vi "WSVCAP SHL Host LL Interface Core.vi"(0 "Message In":string, 11 "error in":errorcluster, 12 "Log (T)":bool=TRUE, 13 "Function":T5, 14 "FPGA":T1) -> (3 "System":T2={"Settings"={"I2C Slave Address"=144, "I2C Clock Rate (Hz)"=20.0, "SPI Clock Rate (Hz)"=50000.0, "RFFE Slave Address"=255, "RFFE Clock Rate (Hz)"=20.0, "Simulate FPGA"=TRUE, "C1 Cap DAC Default"=165, "C2 Cap DAC Default"=165, "C3 Cap DAC Default"=134, "C4 Cap DAC Default"=150}, "FPGA Resource"="", "Online"=FALSE, "I2C Wait Ticks"=0, "SPI Wait Ticks"=0, "RFFE Wait Ticks"=0, "FPGA VI Reference (FPGA Mode)"=refnum, "FPGA VI Reference (Sim Mode)"=refnum} {"Settings"."C4 Cap DAC Default" format="0x%02x"; "Settings"."C3 Cap DAC Default" format="0x%02x"; "Settings"."C2 Cap DAC Default" format="0x%02x"; "Settings"."C1 Cap DAC Default" format="0x%02x"; "Settings"."RFFE Clock Rate (Hz)" format="%.0f Hz"; "Settings"."RFFE Slave Address" format="0x%02x"; "Settings"."I2C Clock Rate (Hz)" format="%.0f Hz"; "Settings"."SPI Clock Rate (Hz)" format="%.0f Hz"; "Settings"."I2C Slave Address" format="0x%02x"}, 4 "Message Out":string, 15 "error out":errorcluster)   [LabVIEW 2017]
uses:
  Type Defs/WSVCAP SHL Function Enum.ctl
  Type Defs/WSVCAP SHL Core System Cluster.ctl
  Type Defs/WSVCAP SHL I2C Settings Cluster.ctl
  Type Defs/WSVCAP SHL FPGA Ref.ctl
  Type Defs/WSVCAP SHL FPGA Enum.ctl
  user.lib/Utilities/Type Defs/MISC IO Choice Enum.ctl
  Type Defs/WSVCAP SHL Gatekeeper Operation Enum.ctl
  user.lib/Configuration Files/Type Defs/CFG File Operation Enum.ctl
  Type Defs/WSVCAP SHL Top Level Control Enum.ctl
  <vilib>/FPGAPlugInAG/PXI-7813R/niLvFpga_Open_PXI-7813R.vi
  <vilib>/FPGAPlugInAG/PXI-7813R/niLvFpga_Reset_PXI-7813R.vi
  <vilib>/FPGAPlugInAG/PXI-7813R/niLvFpga_Run_PXI-7813R.vi
  <vilib>/FPGAPlugInAG/PXI-7813R/niLvFpga_Abort_PXI-7813R.vi
  <vilib>/FPGAPlugInAG/PXI-7813R/niLvFpga_Close_PXI-7813R.vi
  <vilib>/rvi/interface/nirviOpenFPGA/nirviOpenFPGA.xnode
  FPGA Bitfiles/WSVCAPShell_WiSpryFPGA1_WSVCAPSHLFPGATLT_ffr+nD2N+rA.lvbitx
  <vilib>/rvi/interface/nirviMethod/nirviMethod.xnode
  <vilib>/rvi/interface/nirviCloseFPGA/nirviCloseFPGA.xnode
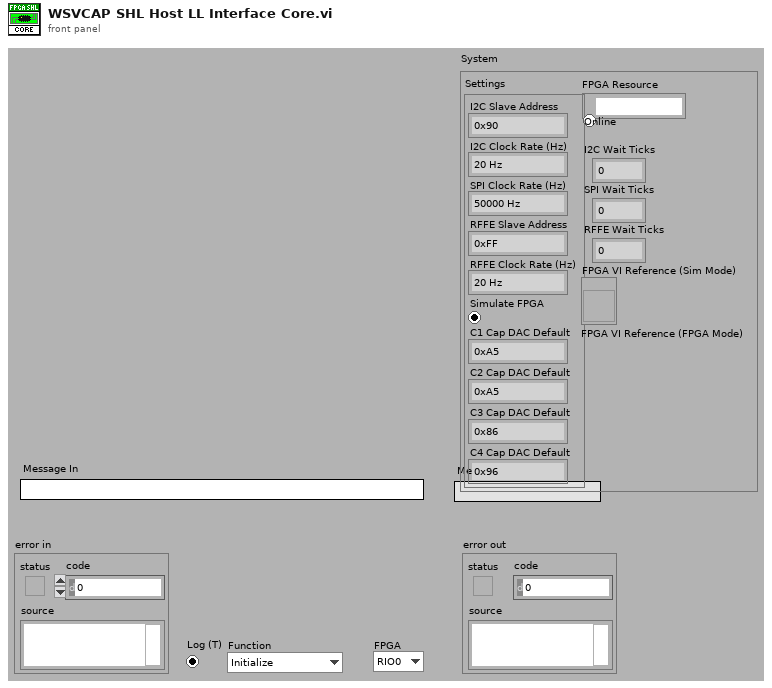
[diagram p1: front panel]
types:
  T1 = typedef "WSVCAP SHL FPGA Enum.ctl" = enum16{"RIO0", "RIO1"}
  T2 = typedef "WSVCAP SHL Core System Cluster.ctl" = cluster{"Settings":T3, "FPGA Resource":tag, "Online":bool, "I2C Wait Ticks":u32, "SPI Wait Ticks":u32, "RFFE Wait Ticks":u32, "FPGA VI Reference (FPGA Mode)":T4, "FPGA VI Reference (Sim Mode)":refnum<vi>}
  T3 = typedef "WSVCAP SHL I2C Settings Cluster.ctl" = cluster{"I2C Slave Address":u8, "I2C Clock Rate (Hz)":dbl, "SPI Clock Rate (Hz)":dbl, "RFFE Slave Address":u8, "RFFE Clock Rate (Hz)":dbl, "Simulate FPGA":bool, "C1 Cap DAC Default":u8, "C2 Cap DAC Default":u8, "C3 Cap DAC Default":u8, "C4 Cap DAC Default":u8}
  T4 = typedef "WSVCAP SHL FPGA Ref.ctl" = refnum<k20>
  T5 = typedef "WSVCAP SHL Function Enum.ctl" = enum16{"Initialize", "Configure I2C", "Configure RFFE", "Write I2C", "Read I2C", "Write RFFE", "Read RFFE", "Start RFFE Cycle", "Stop RFFE Cycle", "Get Status", "Close"}
  T6 = typedef "WSVCAP SHL Gatekeeper Operation Enum.ctl" = enum16{"Initialize", "Lock", "Unlock", "Close"}
  T7 = typedef "MISC IO Choice Enum.ctl" = enum16{"Read", "Write"}
  T8 = typedef "CFG File Operation Enum.ctl" = enum16{"Read", "Write", "Copy", "Edit"}
  T9 = enum32{"Invalid", "Standard", "Closed", "Hidden", "Minimized", "Maximized"}
  T10 = typedef "WSVCAP SHL Top Level Control Enum.ctl" = enum16{"Start", "Cmd", "Transaction", "Wait Ticks", "Socket Mask", "UUT Set", "Slave Address", "Sub Address", "Bytes to Write", "Bytes to Read", "Write Data", "Write Flag", "Read Data", "Read Flag", "Ack Read", "Read Status Flag", "Ack Read Status", "Status", "Cycle Count", "Stop Cycle", "Exit"}
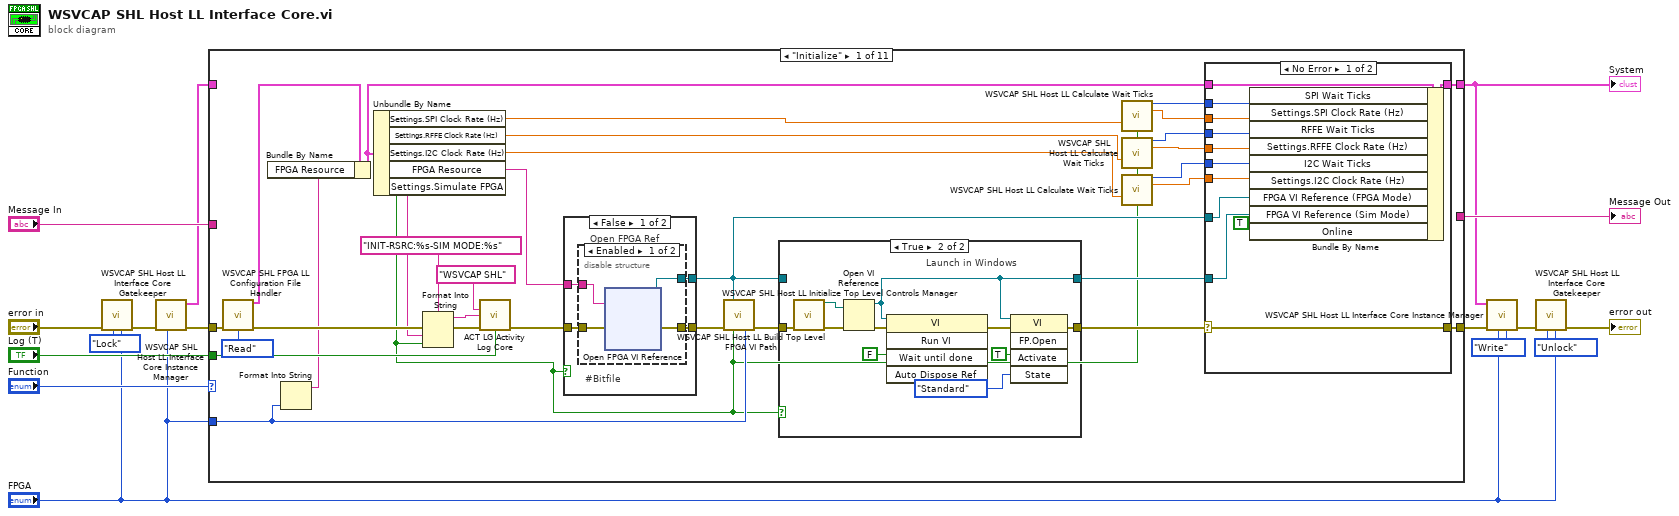
[diagram p0: block diagram]
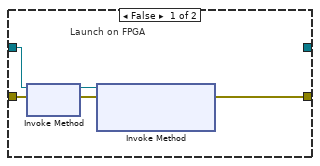
[diagram p4: hidden frame]
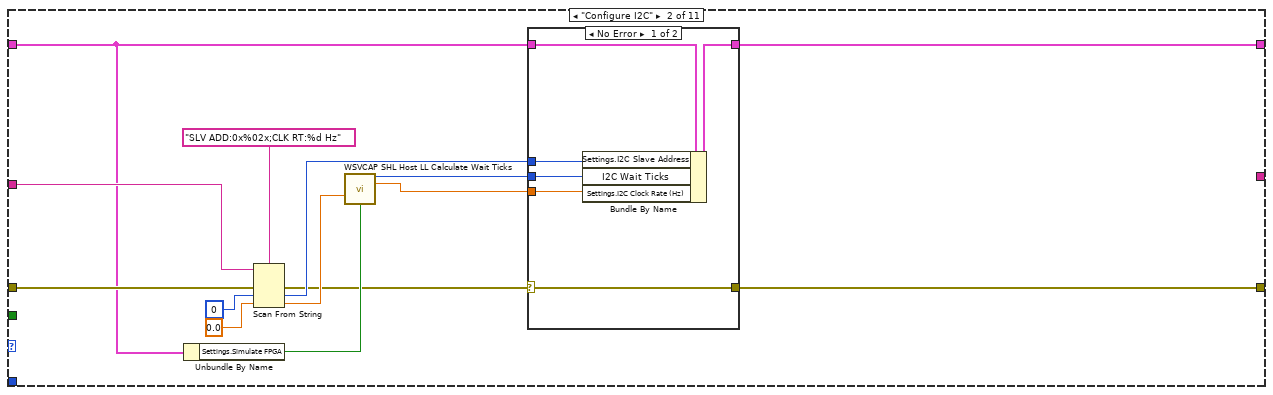
[diagram p6: hidden frame]
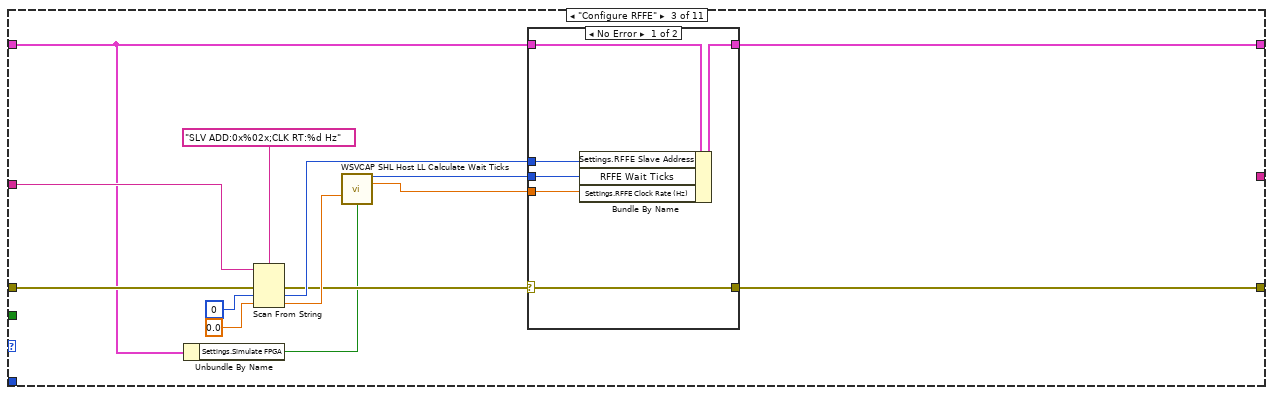
[diagram p8: hidden frame]
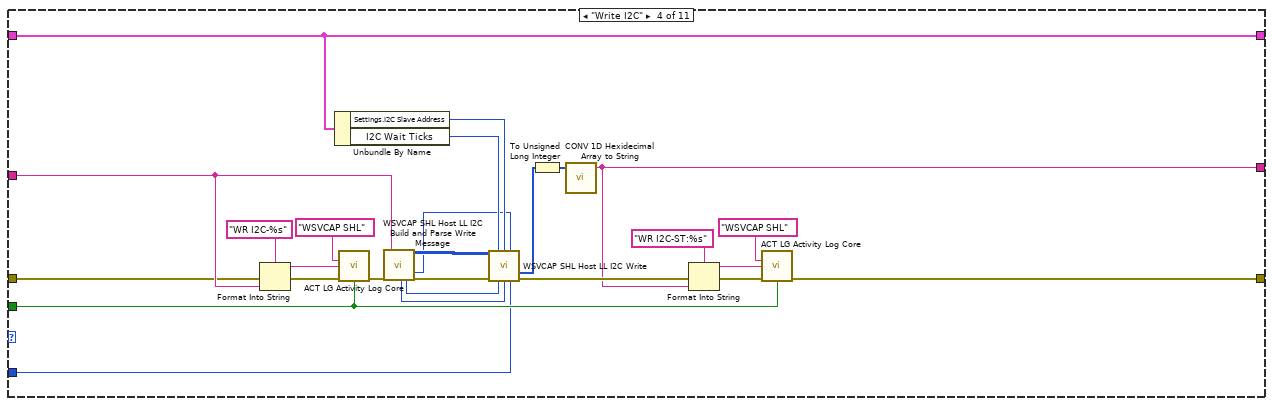
[diagram p10: hidden frame]
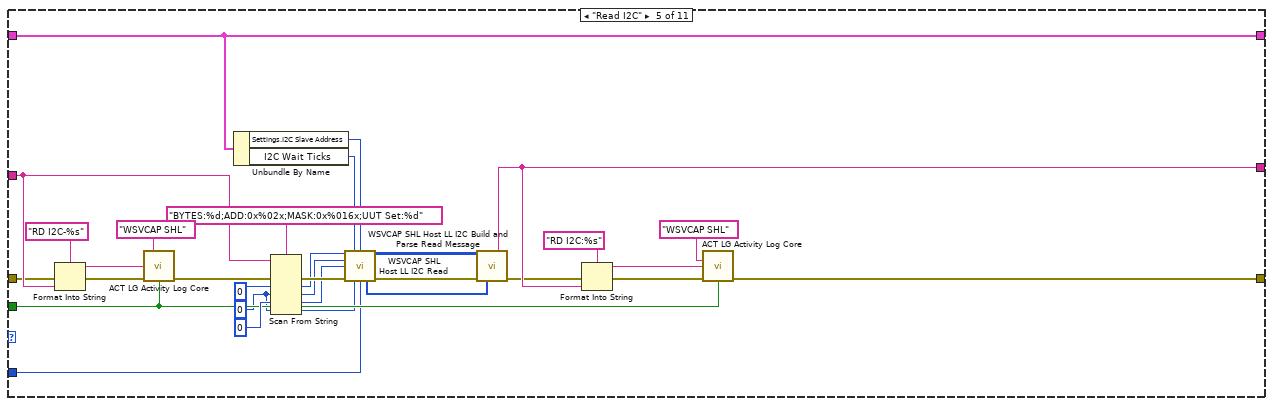
[diagram p11: hidden frame]
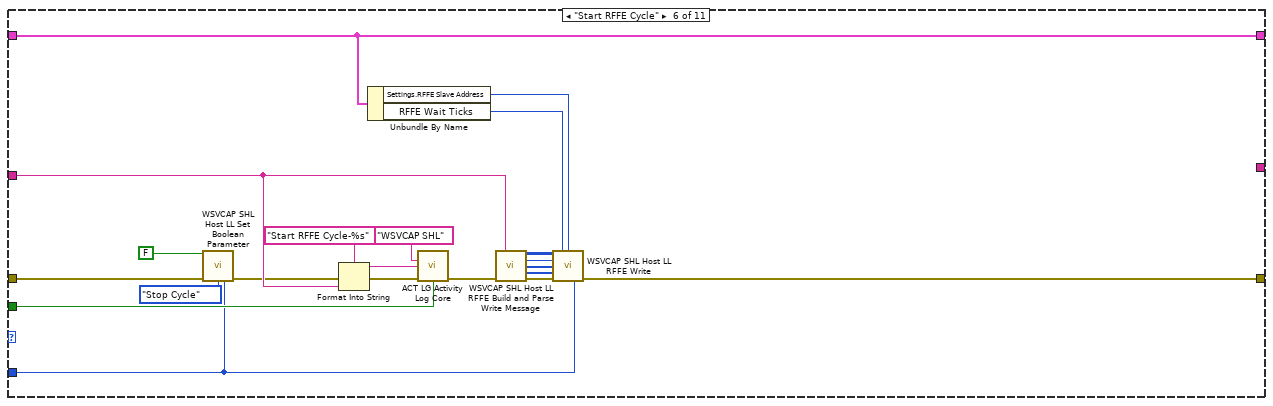
[diagram p12: hidden frame]
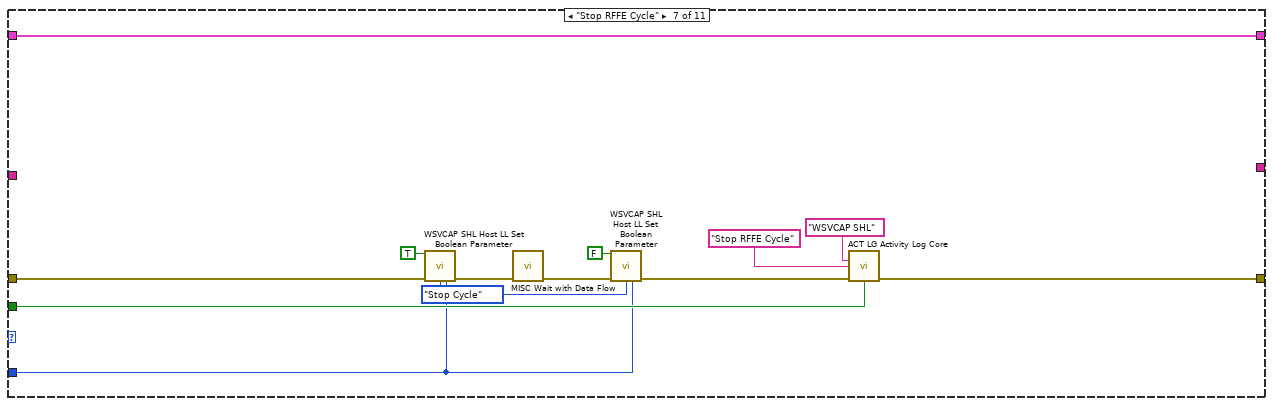
[diagram p13: hidden frame]
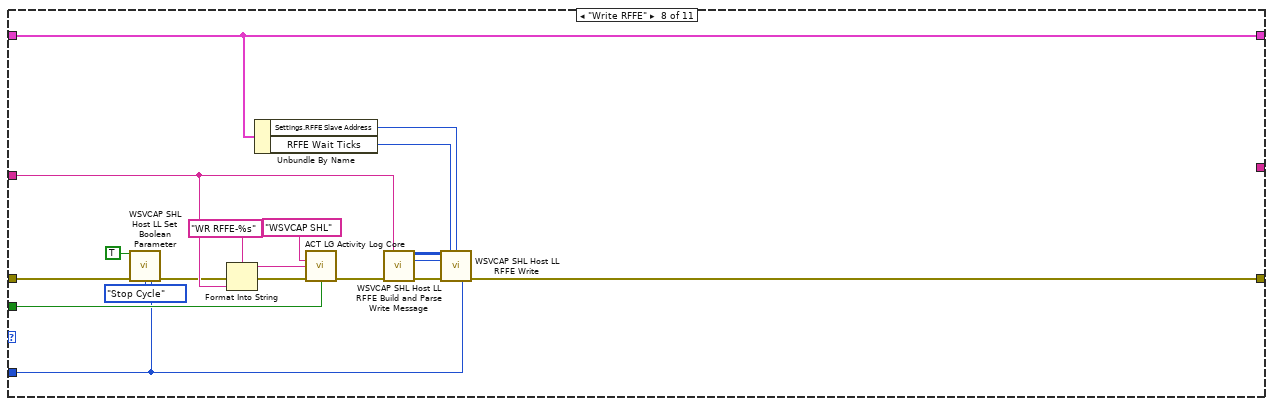
[diagram p14: hidden frame]
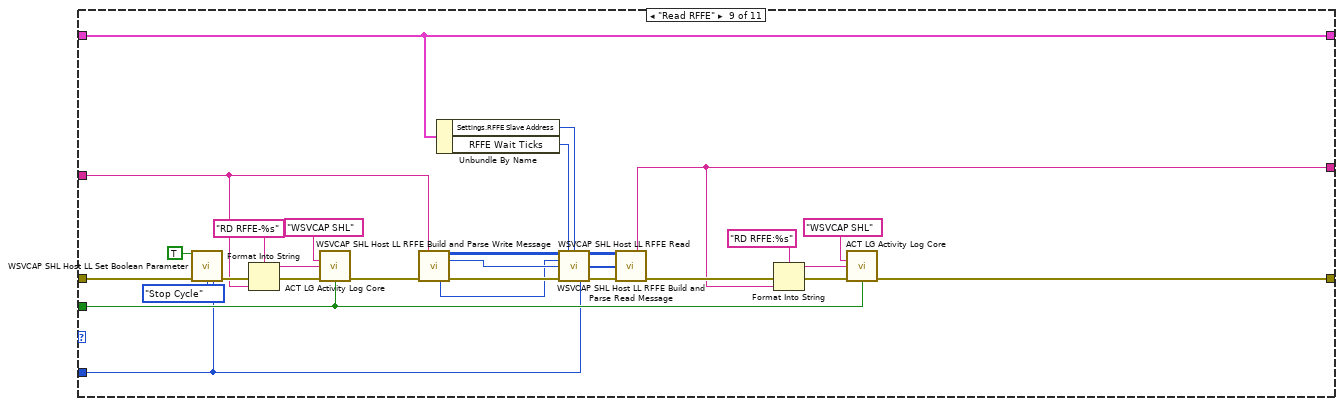
[diagram p15: hidden frame]
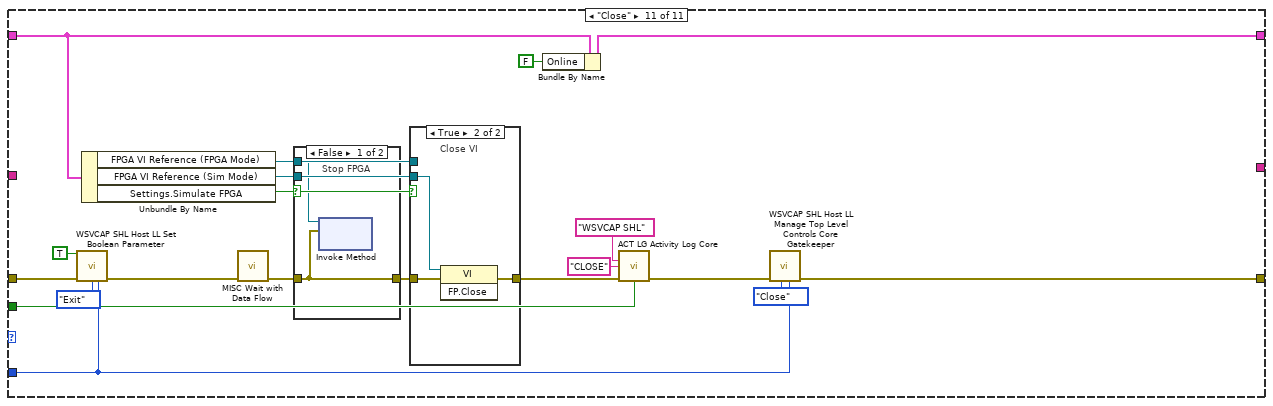
[diagram p17: hidden frame]
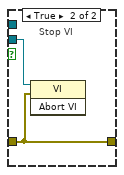
[diagram p18: hidden frame]
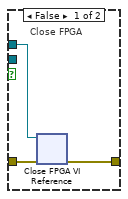
[diagram p19: hidden frame]
diagram:
  n1 = call "WSVCAP SHL Host LL Interface Core Gatekeeper.vi"("FPGA"="FPGA", "Operation"=WSVCAP_SHL_Gatekeeper_Operation_Enum."Lock", "error in (no error)"="error in") -> ("error out"=w4:errorcluster)  [unwired: 8 in]
  n2 = call "WSVCAP SHL Host LL Interface Core Instance Manager.vi"("FPGA"="FPGA", "error in (no error)"=w4) -> ("error out"=w10:errorcluster, "FGPA Interface Out"=w9:T2)  [unwired: 8 in]
  n3 = case shown="\"Initialize\"" "Function" {
    tunnel: w10 -> [w43 w98 w120 w149 w170 w190 w216 w230 w253 w270 w288]
    tunnel: "Message In" -> [_ w97 w119 w150 w171 w201 _ w233 w246 _ _]
    tunnel: [w46 w99 w121 w151 w167 w199 w219 w225 w257 w270 w273] -> w12
    tunnel: [w47 w100 w122 w137 w163 w195 w221 w227 w251 w271 w291] -> w11
    tunnel: w9 -> [_ w93 w115 w137 w163 w195 w221 w227 w251 w271 w281]
    tunnel: [_ _ _ w141 w172 _ _ _ w256 _ _] -> w14
    tunnel: "Log (T)" -> [w36 _ _ w138 w164 w200 w218 w232 w255 _ w284]
    tunnel: "FPGA" -> [w20 _ _ w132 w158 w188 w214 w223 w242 _ w272]
    frame "Initialize" {
      n4 = call "WSVCAP SHL FPGA LL Configuration File Handler.vi"("Error In (no error)"=w43, "Operation"=CFG_File_Operation_Enum."Read") -> ("Object Cluster Out"=w23:T2, "Error Out"=w41:errorcluster)  [unwired: 11 in, 1 out]
      n5 = Format Into String(w20) -> (resulting string=w24:string)  [unwired: 3 in, 1 out]
      n6 = Bundle By Name(cluster=w23, "FPGA Resource"=w24) -> (w22:T2)
      n7 = Unbundle By Name(w22) -> ("Settings.SPI Clock Rate (Hz)"=w31:dbl, "Settings.RFFE Clock Rate (Hz)"=w34:dbl, "Settings.I2C Clock Rate (Hz)"=w38:dbl, "FPGA Resource"=w28:tag, "Settings.Simulate FPGA"=w19:bool)
      n8 = Format Into String(format string="INIT-RSRC:%s-SIM MODE:%s", error in=w41, w28, w19) -> (resulting string=w42:string, error out=w40:errorcluster)  [unwired: 1 in]
      n9 = call "ACT LG Activity Log Core.vi"("Source"="WSVCAP SHL", "Log Line"=w42, "Error In (no error)"=w40, "Log (T)"=w36) -> ("Error Out"=w27:errorcluster)  [unwired: 10 in, 1 out]
      n10 = case shown="False" w19 {
        tunnel: [w51 w57] -> w18
        tunnel: w27 -> [w50 w57]
        tunnel: [w49 _] -> w21
        tunnel: w28 -> [w48 _]
        frame False {
          # "#Bitfile"
          # "Open FPGA Ref"
          n11 = disable-structure shown="Enabled" {
            disable-tunnel: w50 -> [w55 w56]
            disable-tunnel: [w54 w56] -> w51
            disable-tunnel: [w53 _] -> w49
            disable-tunnel: w48 -> [w52 _]
            frame Enabled {
              n12 = xnode "Open FPGA VI Reference"("error in"=w55, "resource name"=w52) -> ("FPGA VI Reference Out"=w53:T4, "error out"=w54:errorcluster)
            }
            frame Disabled {
            }
          }
        }
        frame True {
          # "Simulate FPGA"
        }
      }
      n13 = call "WSVCAP SHL Host LL Initialize Top Level Controls Manager.vi"("FPGA VI Reference (Init Only)"=w21, "error in (no error)"=w18, "Simulate FPGA (Init Only)"=w19, "FPGA"=w20) -> ("error out"=w17:errorcluster)  [unwired: 11 in]
      n14 = case shown="True" w19 {
        tunnel: w17 -> [w61 w65]
        tunnel: [w60 w68] -> w26
        tunnel: w21 -> [w58 _]
        tunnel: [_ w69] -> w25
        frame False {
          # "Launch on FPGA"
          n15 = xnode "Invoke Method"("FPGA VI Reference In"=w58, "error in"=w61) -> ("FPGA VI Reference Out"=w59:T4, "error out"=w62:errorcluster)
          n16 = xnode "Invoke Method"("FPGA VI Reference In"=w59, "error in"=w62) -> ("error out"=w60:errorcluster)  [unwired: 1 in, 1 out]
        }
        frame True {
          # "Launch in Windows"
          n17 = call "WSVCAP SHL Host LL Build Top Level FPGA VI Path.vi"("Error In (no error)"=w65) -> ("Top Level FPGA VI Path"=w63:path, "Error Out"=w64:errorcluster)  [unwired: 13 in]
          n18 = Open VI Reference(vi path=w63, error in (no error)=w64) -> (vi reference=w69:refnum<vi>, error out=w72:errorcluster)  [unwired: 4 in]
          n19 = invoke class="VI" method="Run VI"(reference=w69, error in=w72, "Wait until done"=FALSE ("Wait Until Done")) -> (error out=w70:errorcluster)  [unwired: 2 in, 4 out]
          n20 = invoke class="VI" method="FP.Open"(reference=w69, error in=w70, "Activate"=TRUE ("Activate?"), "State"=T9."Standard" ("Front Panel Window:State")) -> (error out=w68:errorcluster)  [unwired: 1 in, 4 out]
        }
      }
      n21 = call "WSVCAP SHL Host LL Calculate Wait Ticks.vi"("Clock Rate (Hz)"=w31, "Simulate FPGA"=w19) -> ("Wait Ticks"=w30:u32, "Actual Rate (Hz)"=w29:dbl)  [unwired: 12 in]
      n22 = call "WSVCAP SHL Host LL Calculate Wait Ticks.vi"("Clock Rate (Hz)"=w34, "Simulate FPGA"=w19) -> ("Wait Ticks"=w33:u32, "Actual Rate (Hz)"=w32:dbl)  [unwired: 12 in]
      n23 = call "WSVCAP SHL Host LL Calculate Wait Ticks.vi"("Clock Rate (Hz)"=w38, "Simulate FPGA"=w19) -> ("Wait Ticks"=w35:u32, "Actual Rate (Hz)"=w45:dbl)  [unwired: 12 in]
      n24 = case shown="No Error" w26 {
        selector: w26 -> [w82 w85]
        tunnel: w22 -> [w84 w86]
        tunnel: [w83 w86] -> w47
        tunnel: [w82 w85] -> w46
        tunnel: w45 -> [w81 _]
        tunnel: w35 -> [w80 _]
        tunnel: w33 -> [w79 _]
        tunnel: w32 -> [w78 _]
        tunnel: w30 -> [w77 _]
        tunnel: w29 -> [w76 _]
        tunnel: w21 -> [w74 _]
        tunnel: w25 -> [w73 _]
        frame No Error {
          n25 = Bundle By Name(cluster=w84, "SPI Wait Ticks"=w77, "Settings.SPI Clock Rate (Hz)"=w76, "RFFE Wait Ticks"=w79, "Settings.RFFE Clock Rate (Hz)"=w78, "I2C Wait Ticks"=w80, "Settings.I2C Clock Rate (Hz)"=w81, "FPGA VI Reference (FPGA Mode)"=w74, "FPGA VI Reference (Sim Mode)"=w73, "Online"=TRUE) -> (w83:T2)
        }
        frame Error {
        }
      }
    }
    frame "Configure I2C" {
      n26 = Unbundle By Name(w93) -> ("Settings.Simulate FPGA"=w92:bool)
      n27 = Scan From String(format string="SLV ADD:0x%02x;CLK RT:%d Hz", input string=w97, error in=w98, default 1=u8 0 ("I2C_Slave Address"), default 2=0.0 ("Clock Rate (Hz)")) -> (error out=w87:errorcluster, output 1=w94:u8, output 2=w90:dbl)  [unwired: 1 in, 2 out]
      n28 = call "WSVCAP SHL Host LL Calculate Wait Ticks.vi"("Clock Rate (Hz)"=w90, "Simulate FPGA"=w92) -> ("Wait Ticks"=w88:u32, "Actual Rate (Hz)"=w89:dbl)  [unwired: 12 in]
      n29 = case shown="No Error" w87 {
        selector: w87 -> [w104 w107]
        tunnel: w93 -> [w106 w108]
        tunnel: [w105 w108] -> w100
        tunnel: [w104 w107] -> w99
        tunnel: w94 -> [w103 _]
        tunnel: w89 -> [w102 _]
        tunnel: w88 -> [w101 _]
        frame No Error {
          n30 = Bundle By Name(cluster=w106, "Settings.I2C Slave Address"=w103, "I2C Wait Ticks"=w101, "Settings.I2C Clock Rate (Hz)"=w102) -> (w105:T2)
        }
        frame Error {
        }
      }
    }
    frame "Configure RFFE" {
      n31 = Unbundle By Name(w115) -> ("Settings.Simulate FPGA"=w109:bool)
      n32 = Scan From String(format string="SLV ADD:0x%02x;CLK RT:%d Hz", input string=w119, error in=w120, default 1=u8 0 ("I2C_Slave Address"), default 2=0.0 ("Clock Rate (Hz)")) -> (error out=w110:errorcluster, output 1=w116:u8, output 2=w113:dbl)  [unwired: 1 in, 2 out]
      n33 = call "WSVCAP SHL Host LL Calculate Wait Ticks.vi"("Clock Rate (Hz)"=w113, "Simulate FPGA"=w109) -> ("Wait Ticks"=w112:u32, "Actual Rate (Hz)"=w111:dbl)  [unwired: 12 in]
      n34 = case shown="No Error" w110 {
        selector: w110 -> [w126 w129]
        tunnel: w115 -> [w128 w130]
        tunnel: [w127 w130] -> w122
        tunnel: [w126 w129] -> w121
        tunnel: w116 -> [w125 _]
        tunnel: w111 -> [w124 _]
        tunnel: w112 -> [w123 _]
        frame No Error {
          n35 = Bundle By Name(cluster=w128, "Settings.RFFE Slave Address"=w125, "RFFE Wait Ticks"=w123, "Settings.RFFE Clock Rate (Hz)"=w124) -> (w127:T2)
        }
        frame Error {
        }
      }
    }
    frame "Write I2C" {
      n36 = Format Into String(format string="WR I2C-%s", error in=w149, w150) -> (resulting string=w146:string, error out=w148:errorcluster)  [unwired: 1 in]
      n37 = Unbundle By Name(w137) -> ("Settings.I2C Slave Address"=w134:u8, "I2C Wait Ticks"=w136:u32)
      n38 = call "ACT LG Activity Log Core.vi"("Source"="WSVCAP SHL", "Log Line"=w146, "Error In (no error)"=w148, "Log (T)"=w138) -> ("Error Out"=w153:errorcluster)  [unwired: 10 in, 1 out]
      n39 = call "WSVCAP SHL Host LL I2C Build and Parse Write Message.vi"("error in"=w153, "Message In"=w150) -> ("UUT Set (0/1) Out (Legacy)"=w133:u8, "Sub Address Out"=w135:u8, "C Write Data Out [DUT Ordered]"=w155:u8[][], "Socket Mask [U64] Out"=w131:u64, "error out"=w156:errorcluster)  [unwired: 12 in, 1 out]
      n40 = call "WSVCAP SHL Host LL I2C Write.vi"("C1 Data Out [DUT Ordered]"=w155, "Wait Ticks"=w136, "Slave Address"=w134, "Socket Mask [U64]"=w131, "error in"=w156, "Sub Address"=w135, "UUT Set (0/1)"=w133, "FPGA"=w132) -> ("Status"=w143:u8[], "error out"=w145:errorcluster)  [unwired: 6 in]
      n41 = To Unsigned Long Integer(number=w143) -> (unsigned 32bit integer=w142:u32[])
      n42 = call "CONV 1D Hexidecimal Array to String.vi"("1-D Hexidecimal"=w142) -> ("String"=w141:string)  [unwired: 8 in]
      n43 = Format Into String(format string="WR I2C-ST:%s", error in=w145, w141) -> (resulting string=w139:string, error out=w144:errorcluster)  [unwired: 1 in]
      n44 = call "ACT LG Activity Log Core.vi"("Source"="WSVCAP SHL", "Log Line"=w139, "Error In (no error)"=w144, "Log (T)"=w138) -> ("Error Out"=w151:errorcluster)  [unwired: 10 in, 1 out]
    }
    frame "Read I2C" {
      w160 = u8 0 ("Sub Address [U8]")
      n45 = Format Into String(format string="RD I2C-%s", error in=w170, w171) -> (resulting string=w176:string, error out=w178:errorcluster)  [unwired: 1 in]
      n46 = call "ACT LG Activity Log Core.vi"("Source"="WSVCAP SHL", "Log Line"=w176, "Error In (no error)"=w178, "Log (T)"=w164) -> ("Error Out"=w169:errorcluster)  [unwired: 10 in, 1 out]
      n47 = Unbundle By Name(w163) -> ("Settings.I2C Slave Address"=w161:u8, "I2C Wait Ticks"=w162:u32)
      n48 = Scan From String(format string="BYTES:%d;ADD:0x%02x;MASK:0x%016x;UUT Set:%d", input string=w171, error in=w169, default 1=u8 0 ("Bytes to Read"), default 2=w160, default 3=u64 0 ("Socket Mask [U32]"), default 4=w160) -> (error out=w187:errorcluster, output 1=w184:u8, output 2=w182:u8, output 3=w183:u64, output 4=w159:u8)  [unwired: 1 in, 2 out]
      n49 = call "WSVCAP SHL Host LL I2C Read.vi"("Bytes to Read"=w184, "Wait Ticks"=w162, "Slave Address"=w161, "Sub Address [U8]"=w182, "Socket Mask [U64]"=w183, "error in"=w187, "UUT Set (0/1)"=w159, "FPGA"=w158) -> ("C1:1-12 Read Data"=w180:u8[][], "Status"=w157:u8[], "error out"=w181:errorcluster)  [unwired: 5 in]
      n50 = call "WSVCAP SHL Host LL I2C Build and Parse Read Message.vi"("C1 Read Data In"=w180, "error in"=w181, "Status In"=w157) -> ("Message Out"=w172:string, "error out"=w168:errorcluster)  [unwired: 9 in, 2 out]
      n51 = Format Into String(format string="RD I2C:%s", error in=w168, w172) -> (resulting string=w173:string, error out=w175:errorcluster)  [unwired: 1 in]
      n52 = call "ACT LG Activity Log Core.vi"("Source"="WSVCAP SHL", "Log Line"=w173, "Error In (no error)"=w175, "Log (T)"=w164) -> ("Error Out"=w167:errorcluster)  [unwired: 10 in, 1 out]
    }
    frame "Start RFFE Cycle" {
      n53 = call "WSVCAP SHL Host LL Set Boolean Parameter.vi"("Boolean In"=FALSE ("Cycle (F:Write/Read - T:Write Only - No Read)"), "error in (no error)"=w190, "FPGA Top Level Control"=WSVCAP_SHL_Top_Level_Control_Enum."Stop Cycle", "FPGA"=w188) -> ("error out"=w189:errorcluster)  [unwired: 11 in]
      n54 = Format Into String(format string="Start RFFE Cycle-%s", error in=w189, w201) -> (resulting string=w203:string, error out=w205:errorcluster)  [unwired: 1 in]
      n55 = Unbundle By Name(w195) -> ("Settings.RFFE Slave Address"=w193:u8, "RFFE Wait Ticks"=w194:u32)
      n56 = call "ACT LG Activity Log Core.vi"("Source"="WSVCAP SHL", "Log Line"=w203, "Error In (no error)"=w205, "Log (T)"=w200) -> ("Error Out"=w202:errorcluster)  [unwired: 10 in, 1 out]
      n57 = call "WSVCAP SHL Host LL RFFE Build and Parse Write Message.vi"("Message In"=w201, "error in"=w202) -> ("Write Data Out [DUT Ordered]"=w207:u8[][], "Socket Mask [U16] Out"=w198:u64, "Cycle CMD Lengths Out (bits)"=w197:u8[], "Cycle CMD Delay Out (ticks)"=w196:u32[], "error out"=w208:errorcluster)  [unwired: 7 in, 2 out]
      n58 = call "WSVCAP SHL Host LL RFFE Write.vi"("RTFFE Data"=w207, "Wait Ticks"=w194, "Slave Address"=w193, "Socket Mask"=w198, "Cycle CMD Lengths Out (bits)"=w197, "Cycle CMD Delay Out (ticks)"=w196, "error in"=w208, "FPGA"=w188) -> ("error out"=w199:errorcluster)  [unwired: 6 in, 1 out]
    }
    frame "Stop RFFE Cycle" {
      w213 = WSVCAP_SHL_Top_Level_Control_Enum."Stop Cycle" ("FPGA Top Level Control")
      n59 = call "WSVCAP SHL Host LL Set Boolean Parameter.vi"("Boolean In"=TRUE ("Cycle (F:Write/Read - T:Write Only - No Read)"), "error in (no error)"=w216, "FPGA Top Level Control"=w213, "FPGA"=w214) -> ("error out"=w212:errorcluster)  [unwired: 11 in]
      n60 = call "MISC Wait with Data Flow.vi"("Error In (no error)"=w212) -> ("Error Out"=w211:errorcluster)  [unwired: 8 in, 2 out]
      n61 = call "WSVCAP SHL Host LL Set Boolean Parameter.vi"("Boolean In"=FALSE ("Cycle (F:Write/Read - T:Write Only - No Read)"), "error in (no error)"=w211, "FPGA Top Level Control"=w213, "FPGA"=w214) -> ("error out"=w215:errorcluster)  [unwired: 11 in]
      n62 = call "ACT LG Activity Log Core.vi"("Source"="WSVCAP SHL", "Log Line"="Stop RFFE Cycle" ("format string"), "Error In (no error)"=w215, "Log (T)"=w218) -> ("Error Out"=w219:errorcluster)  [unwired: 10 in, 1 out]
    }
    frame "Write RFFE" {
      n63 = call "WSVCAP SHL Host LL Set Boolean Parameter.vi"("Boolean In"=TRUE ("Cycle (F:Write/Read - T:Write Only - No Read)"), "error in (no error)"=w230, "FPGA Top Level Control"=WSVCAP_SHL_Top_Level_Control_Enum."Stop Cycle", "FPGA"=w223) -> ("error out"=w229:errorcluster)  [unwired: 11 in]
      n64 = Format Into String(format string="WR RFFE-%s", error in=w229, w233) -> (resulting string=w235:string, error out=w237:errorcluster)  [unwired: 1 in]
      n65 = Unbundle By Name(w227) -> ("Settings.RFFE Slave Address"=w224:u8, "RFFE Wait Ticks"=w226:u32)
      n66 = call "ACT LG Activity Log Core.vi"("Source"="WSVCAP SHL", "Log Line"=w235, "Error In (no error)"=w237, "Log (T)"=w232) -> ("Error Out"=w234:errorcluster)  [unwired: 10 in, 1 out]
      n67 = call "WSVCAP SHL Host LL RFFE Build and Parse Write Message.vi"("Message In"=w233, "error in"=w234) -> ("Write Data Out [DUT Ordered]"=w239:u8[][], "Socket Mask [U16] Out"=w228:u64, "error out"=w240:errorcluster)  [unwired: 7 in, 4 out]
      n68 = call "WSVCAP SHL Host LL RFFE Write.vi"("RTFFE Data"=w239, "Wait Ticks"=w226, "Slave Address"=w224, "Socket Mask"=w228, "error in"=w240, "FPGA"=w223) -> ("error out"=w225:errorcluster)  [unwired: 8 in, 1 out]
    }
    frame "Read RFFE" {
      n69 = call "WSVCAP SHL Host LL Set Boolean Parameter.vi"("Boolean In"=TRUE ("Cycle (F:Write/Read - T:Write Only - No Read)"), "error in (no error)"=w253, "FPGA Top Level Control"=WSVCAP_SHL_Top_Level_Control_Enum."Stop Cycle", "FPGA"=w242) -> ("error out"=w252:errorcluster)  [unwired: 11 in]
      n70 = Format Into String(format string="RD RFFE-%s", error in=w252, w246) -> (resulting string=w262:string, error out=w264:errorcluster)  [unwired: 1 in]
      n71 = call "ACT LG Activity Log Core.vi"("Source"="WSVCAP SHL", "Log Line"=w262, "Error In (no error)"=w264, "Log (T)"=w255) -> ("Error Out"=w248:errorcluster)  [unwired: 10 in, 1 out]
      n72 = call "WSVCAP SHL Host LL RFFE Build and Parse Write Message.vi"("Message In"=w246, "error in"=w248) -> ("Write Data Out [DUT Ordered]"=w245:u8[][], "Socket Mask [U16] Out"=w244:u64, "Byte Count"=w243:u8, "error out"=w247:errorcluster)  [unwired: 7 in, 3 out]
      n73 = Unbundle By Name(w251) -> ("Settings.RFFE Slave Address"=w249:u8, "RFFE Wait Ticks"=w250:u32)
      n74 = call "WSVCAP SHL Host LL RFFE Read.vi"("RFFE Data [DUT Ordered]"=w245, "Wait Ticks"=w250, "Slave Address"=w249, "Bytes to Read"=w243, "Socket Mask [U64]"=w244, "error in"=w247, "FPGA"=w242) -> ("RFFE Read Data [DUT Ordered]"=w268:u8[][], "Status"=w267:u8[], "error out"=w269:errorcluster)  [unwired: 6 in]
      n75 = call "WSVCAP SHL Host LL RFFE Build and Parse Read Message.vi"("Write Data In"=w268, "Status In"=w267, "error in"=w269) -> ("Message Out"=w256:string, "error out"=w258:errorcluster)  [unwired: 9 in, 2 out]
      n76 = Format Into String(format string="RD RFFE:%s", error in=w258, w256) -> (resulting string=w259:string, error out=w261:errorcluster)  [unwired: 1 in]
      n77 = call "ACT LG Activity Log Core.vi"("Source"="WSVCAP SHL", "Log Line"=w259, "Error In (no error)"=w261, "Log (T)"=w255) -> ("Error Out"=w257:errorcluster)  [unwired: 10 in, 1 out]
    }
    frame "Get Status" {
    }
    frame "Close" {
      n78 = call "WSVCAP SHL Host LL Set Boolean Parameter.vi"("Boolean In"=TRUE ("Start"), "error in (no error)"=w288, "FPGA Top Level Control"=WSVCAP_SHL_Top_Level_Control_Enum."Exit", "FPGA"=w272) -> ("error out"=w277:errorcluster)  [unwired: 11 in]
      n79 = Unbundle By Name(w281) -> ("FPGA VI Reference (FPGA Mode)"=w280:T4, "FPGA VI Reference (Sim Mode)"=w279:refnum<vi>, "Settings.Simulate FPGA"=w278:bool)
      n80 = call "MISC Wait with Data Flow.vi"("Error In (no error)"=w277) -> ("Error Out"=w282:errorcluster)  [unwired: 8 in, 2 out]
      n81 = case shown="False" w278 {
        tunnel: w280 -> [w293 _]
        tunnel: w282 -> [w292 w294]
        tunnel: [w292 w294] -> w283
        tunnel: w279 -> [_ w295]
        frame False {
          # "Stop FPGA"
          n82 = xnode "Invoke Method"("FPGA VI Reference In"=w293, "error in"=w292) -> ()  [unwired: 2 out]
        }
        frame True {
          # "Stop VI"
          n83 = invoke class="VI" method="Abort VI"(reference=w295, error in=w294) -> ()  [unwired: 1 in, 3 out]
        }
      }
      n84 = case shown="True" w278 {
        tunnel: w283 -> [w298 w301]
        tunnel: w280 -> [w297 _]
        tunnel: [w296 w300] -> w276
        tunnel: w279 -> [_ w299]
        frame False {
          # "Close FPGA"
          n85 = xnode "Close FPGA VI Reference"("FPGA VI Reference In"=w297, "error in"=w298) -> ("error out"=w296:errorcluster)
        }
        frame True {
          # "Close VI"
          n86 = invoke class="VI" method="FP.Close"(reference=w299, error in=w301) -> (error out=w300:errorcluster)  [unwired: 1 in, 2 out]
        }
      }
      n87 = Bundle By Name(cluster=w281, "Online"=FALSE) -> (w291:T2)
      n88 = call "ACT LG Activity Log Core.vi"("Source"="WSVCAP SHL", "Log Line"="CLOSE", "Error In (no error)"=w276, "Log (T)"=w284) -> ("Error Out"=w274:errorcluster)  [unwired: 10 in, 1 out]
      n89 = call "WSVCAP SHL Host LL Manage Top Level Controls Core Gatekeeper.vi"("FPGA"=w272, "Operation"=WSVCAP_SHL_Gatekeeper_Operation_Enum."Close", "error in (no error)"=w274) -> ("error out"=w273:errorcluster)  [unwired: 8 in]
    }
  }
  "Message Out" <- w14
  "System" <- w11
  n90 = call "WSVCAP SHL Host LL Interface Core Instance Manager.vi"("I/O Choice (read)"=MISC_IO_Choice_Enum."Write", "FPGA"="FPGA", "error in (no error)"=w12, "FPGA Interface In"=w11) -> ("error out"=w7:errorcluster)  [unwired: 6 in, 1 out]
  n91 = call "WSVCAP SHL Host LL Interface Core Gatekeeper.vi"("FPGA"="FPGA", "Operation"=WSVCAP_SHL_Gatekeeper_Operation_Enum."Unlock", "error in (no error)"=w7) -> ("error out"=→"error out":errorcluster)  [unwired: 8 in]
